vi "字符串.vi"() -> ()   [LabVIEW 2014]
panel:
  out "数值 3":dbl
  out "数值 2":dbl
  out "数值":dbl
  in  "字符串 2":string
  out "显示 6":string
  in  "旋钮 2":dbl(knob) scale=0.0..10.0
  in  "旋钮":dbl(knob) scale=0.0..10.0
  out "时间标识":timestamp
  out "显示 5":string
  out "显示 4":string
  out "显示 3":string
  out "显示 2":string
  out "姓名长度":i8
  out "显示":string
  in  "字符串":string
  in  "姓名":string
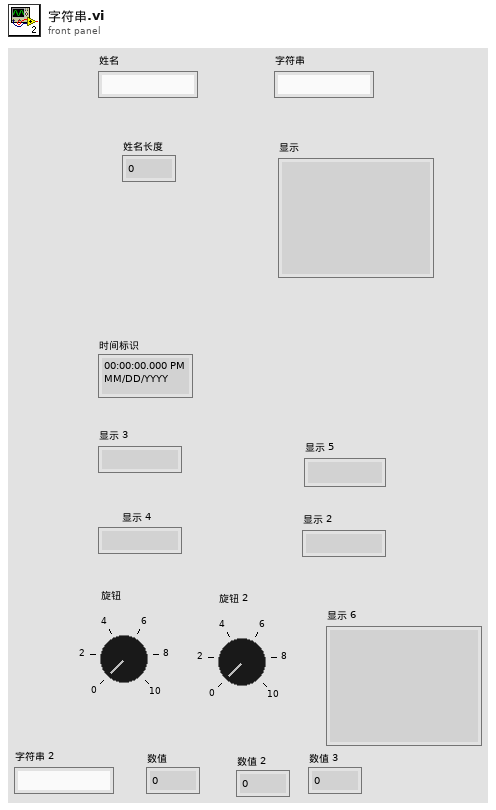
[diagram p1: front panel]
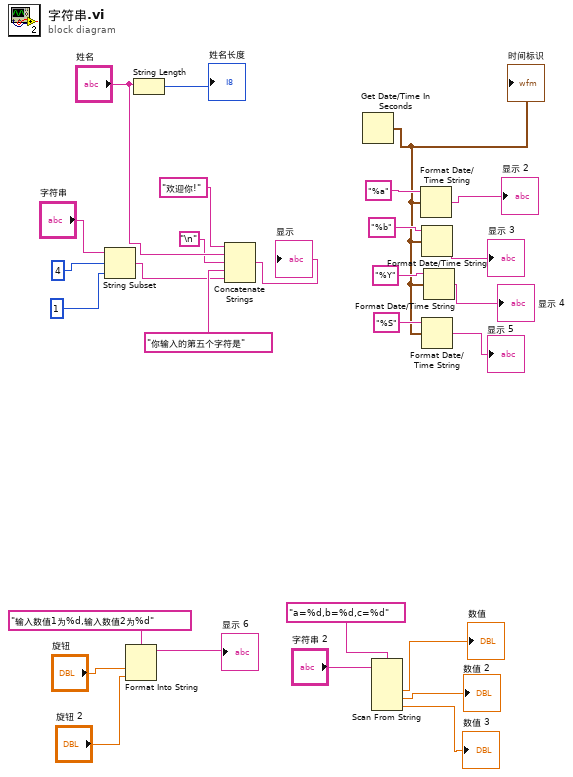
[diagram p0: block diagram]
diagram:
  n1 = String Subset(string="字符串", offset (0)=4, length (rest)=1) -> (substring=w23:string)
  n2 = Format Into String(format string="输入数值1为%d,输入数值2为%d", "旋钮", "旋钮 2") -> (resulting string=→"显示 6":string)  [unwired: 2 in, 1 out]
  n3 = String Length(string="姓名") -> (length=→"姓名长度":i32)
  n4 = Concatenate Strings("欢迎你!", "姓名", "\n", "你输入的第五个字符是", w23) -> (→"显示":string)
  n5 = Get Date/Time In Seconds() -> (seconds since 1Jan1904=w10:timestamp)
  "时间标识" <- w10
  n6 = Scan From String(format string="a=%d,b=%d,c=%d", input string="字符串 2") -> (output 1=→"数值":dbl, output 2=→"数值 2":dbl, output 3=→"数值 3":dbl)  [unwired: 5 in, 3 out]
  n7 = Format Date/Time String(time format string (%c)="%a", seconds (now)=w10) -> (date/time string=→"显示 2":string)  [unwired: 1 in]
  n8 = Format Date/Time String(time format string (%c)="%b", seconds (now)=w10) -> (date/time string=→"显示 3":string)  [unwired: 1 in]
  n9 = Format Date/Time String(time format string (%c)="%S", seconds (now)=w10) -> (date/time string=→"显示 5":string)  [unwired: 1 in]
  n10 = Format Date/Time String(time format string (%c)="%Y", seconds (now)=w10) -> (date/time string=→"显示 4":string)  [unwired: 1 in]
